vi "Arrow_Execute.vi"() -> ()   [LabVIEW 2020]
uses:
  Globals/Arrow_Globals.vi
  Globals/Sensor_Values.vi
panel:
  in  "Kd":dbl
  in  "Ki":dbl
  in  "Kp":dbl
  in  "Earlnator":dbl
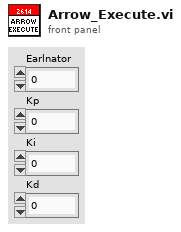
[diagram p1: front panel]
types:
  T1 = typedef "Arrow_Cluster.ctl" = cluster{"Control_States":T2, "Manual_Arrow":dbl, "GoToAngle":bool}
  T2 = typedef "Arrow_Control_States.ctl" = enum16{"No-Op", "Manual_Control", "GoToAngle"}
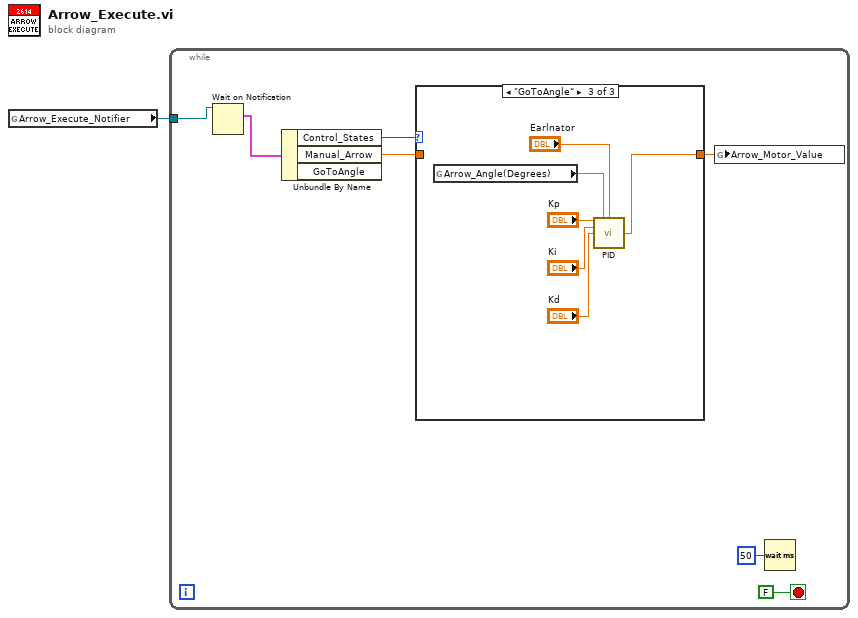
[diagram p0: block diagram]
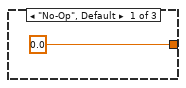
[diagram p2: hidden frame]
diagram:
  n1 = global read "Arrow_Globals.vi" "Arrow_Execute_Notifier"() -> (w1:refnum<notifier>)
  n2 = while {
    tunnel: w1 -> [w8]
    stop <- FALSE stop-if-true
    n3 = Wait on Notification(notifier=w8) -> (notification=w5:T1)  [unwired: 3 in, 3 out]
    n4 = Unbundle By Name(w5) -> ("Control_States"=w4:T2, "Manual_Arrow"=w3:dbl)  [unwired: 1 out]
    n5 = case shown="\"GoToAngle\"" w4 {
      tunnel: [0.0 w10 w11] -> w2
      tunnel: w3 -> [_ w10 _]
      frame "No-Op", Default {
      }
      frame "Manual_Control" {
      }
      frame "GoToAngle" {
        n6 = global read "Sensor_Values.vi" "Arrow_Angle(Degrees)"() -> (w15:dbl)
        n7 = call "PID.vi"("Kp"="Kp", "Process Variable"=w15, "Goal"="Earlnator", "Ki"="Ki", "Kd"="Kd") -> ("Command"=w11:dbl)  [unwired: 8 in, 2 out]
      }
    }
    n8 = global write "Arrow_Globals.vi" "Arrow_Motor_Value"(w2) -> ()
    n9 = Wait (ms)(milliseconds to wait=u32 50) -> ()  [unwired: 1 out]
  }
